vi "Self Alias.vi"(11 "Ex Queue Actor in":refnum<class "Ex Queue Actor.lvclass">) -> (2 "Self Alias":string)   [LabVIEW 2021, in "Ex Queue Actor.lvlib" / "Ex Queue Actor.lvclass"]
uses:
  Ex Queue Actor.lvclass
  Ex Queue Actor.lvclass/Ex Queue Actor.ctl
  Actor/Queue Actor/Queue Actor.lvclass
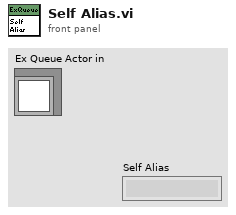
[diagram p1: front panel]
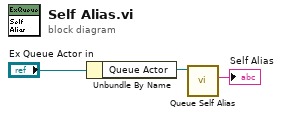
[diagram p0: block diagram]
diagram:
  n1 = Unbundle By Name("Ex Queue Actor in") -> ("Queue Actor"=w1:refnum<class "Queue Actor.lvclass">)
  n2 = call-dynamic "Queue Self Alias.vi"("Actor in"=w1) -> ("Queue Self Alias"=→"Self Alias":string)  [unwired: 10 in]
